vi "ParseChannelList.vi"(8 "error in (no error)":errorcluster, 10 "Channel to Read":T1=enum."AI", 11 "_Property Bundle":cluster{"Name":string, "Value":variant}[](array[cluster])) -> (0 "error out":errorcluster, 2 "Channel Strings":string[](array[string]), 3 "Channel List Out":T2[](array[typedef]))   [LabVIEW 2021]
uses:
  <vilib>/myRIO/Common/Profile Manager Framework/typedefs/Channel Info.ctl
  <vilib>/myRIO/Common/Instrument Driver Framework/Utilities/typedefs/Channel Types.ctl
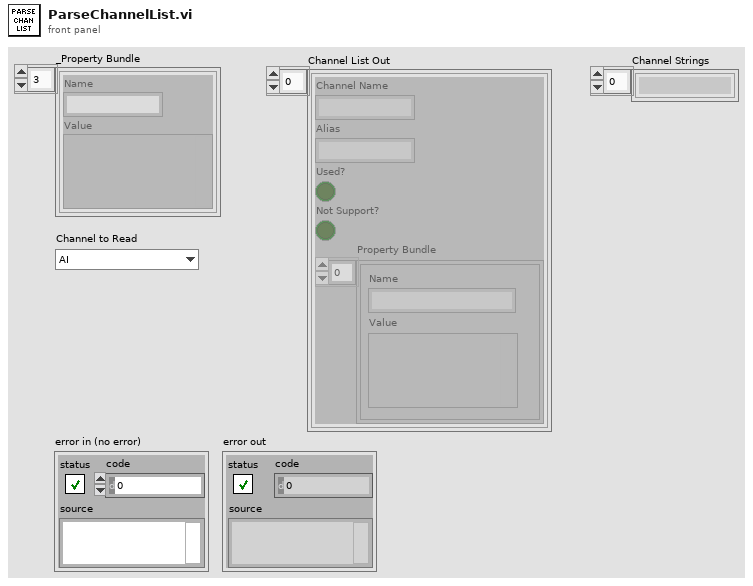
[diagram p1: front panel]
types:
  T1 = typedef "Channel Types.ctl" = enum32{"Unknown", "AI", "AO", "DIO - DI", "DIO", "DIO - DO", "I2C", "PWM", "Encoder", "SPI", "UART", "Accelerometer", "DIO - LED", "DIO - Button", "AI (N Samples)", "AudioIn (N Samples)", "AO (N Samples)", "AudioOut (N Samples)", "DI (N Samples)", "DO (N Samples)", "AI IRQ", "DI IRQ", "Timer IRQ", "RSL", "Relay", "CAN", "AI (Continuous)", "AO (Continuous)"}
  T2 = typedef "Channel Info.ctl" = cluster{"Channel Name":string, "Alias":string, "Used?":bool, "Not Support?":bool, "Property Bundle":cluster{"Name":string, "Value":variant}[]}
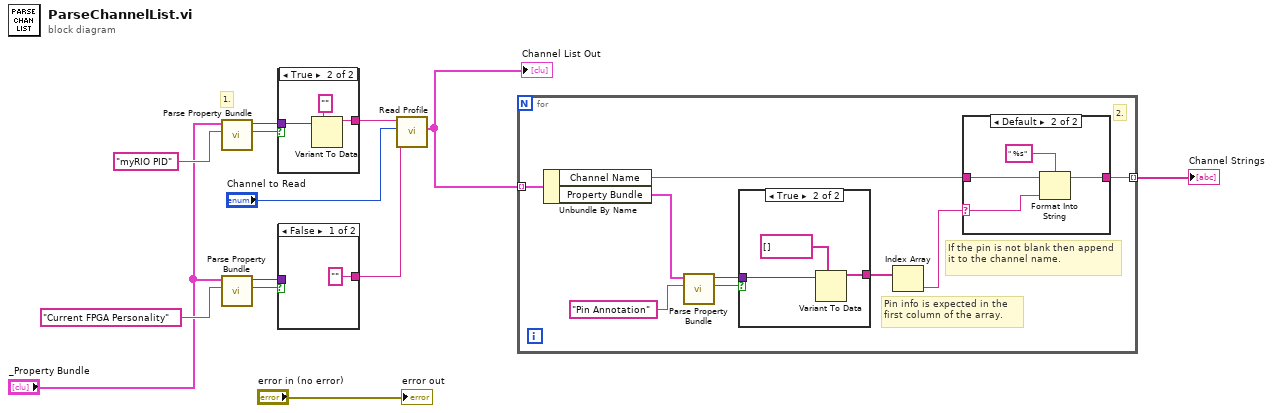
[diagram p0: block diagram]
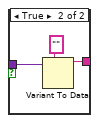
[diagram p2: hidden frame]
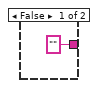
[diagram p3: hidden frame]
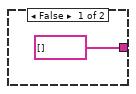
[diagram p4: hidden frame]
diagram:
  # "1."
  n1 = call <vilib>:"Parse Property Bundle.vi"("Name"="myRIO PID", "Property Bundle"="_Property Bundle") -> ("Found?"=w11:bool, "Value"=w10:variant)  [unwired: 8 in]
  n2 = call <vilib>:"Parse Property Bundle.vi"("Name"="Current FPGA Personality", "Property Bundle"="_Property Bundle") -> ("Found?"=w4:bool, "Value"=w5:variant)  [unwired: 8 in]
  n3 = case shown="True" w11 {
    tunnel: w10 -> [_ w17]
    tunnel: ["" ("Name") w15] -> w12
    frame False {
    }
    frame True {
      n4 = Variant To Data(type="" ("Name"), Variant=w17) -> (data=w15:string)  [unwired: 1 in, 1 out]
    }
  }
  n5 = case shown="False" w4 {
    tunnel: w5 -> [_ w21]
    tunnel: ["" ("Name") w19] -> w3
    frame False {
    }
    frame True {
      n6 = Variant To Data(type="" ("Name"), Variant=w21) -> (data=w19:string)  [unwired: 1 in, 1 out]
    }
  }
  n7 = call <vilib>:"Read Profile.vi"("FPGA Name"=w3, "Channel to Read"="Channel to Read", "myRIO PID"=w12) -> ("Channel List Out"=w7:T2[])  [unwired: 7 in, 1 out]
  "Channel List Out" <- w7
  n8 = for {
    tunnel: w7 -> [w29] mode=indexing
    tunnel: [w30] -> w8 mode=indexing
    # "If the pin is not blank then append it to the channel name."
    # "Pin info is expected in the first column of the array."
    # "2."
    n9 = Unbundle By Name(w29) -> ("Channel Name"=w28:string, "Property Bundle"=w27:cluster{"Name":string, "Value":variant}[])
    n10 = call <vilib>:"Parse Property Bundle.vi"("Name"="Pin Annotation", "Property Bundle"=w27) -> ("Found?"=w24:bool, "Value"=w25:variant)  [unwired: 8 in]
    n11 = case shown="True" w24 {
      tunnel: w25 -> [_ w34]
      tunnel: [string[] [] w33] -> w23
      frame False {
      }
      frame True {
        n12 = Variant To Data(type=string[] [], Variant=w34) -> (data=w33:string[])  [unwired: 1 in, 1 out]
      }
    }
    n13 = Index Array(array=w23) -> (element=w22:string)  [unwired: 1 in]
    n14 = case shown="Default" w22 {
      selector: w22 -> [_ w38]
      tunnel: w28 -> [w35 w37]
      tunnel: [w35 w36] -> w30
      frame "" {
      }
      frame Default {
        n15 = Format Into String(format string=" %s", initial string=w37, w38) -> (resulting string=w36:string)  [unwired: 1 in, 1 out]
      }
    }
  }
  "Channel Strings" <- w8
  "error out" <- "error in (no error)"
